vi "HEWH Staged Proportioning Valve Opening.vi"(8 "Error In":errorcluster, 10 "Elapsed Time (sec) in":dbl, 11 "Core HEWH Data Station A":T1 {"Test Patten Setup"."PRAT/RLT Sequence"."Time" format="%<%H:%M:%S>t"; "Test Patten Setup"."Total Gallons Schedule" format="%.2f"}) -> (0 "Error Out":errorcluster, 3 "Prop Valve Setting":dbl)   [LabVIEW 2016]
uses:
  Type Definitions/HEWH Output Information.ctl
  Type Definitions/HEWH Draw Pattern Setup.ctl
  Type Definitions/PRAT Test.ctl
  Utility/Save File/File Setup (Public)/Type Definition/Save File HEWH Heating Control Mode.ctl
  Draw Water Specific/Type Definitions/Terminate Draw Conditions.ctl
  Type Definitions/HEWH Start Conditions.ctl
  Draw Water Specific/Type Definitions/Check Special Condtions.ctl
  Draw Water Specific/Type Definitions/HEWH Special Condition Check.ctl
  Type Definitions/HEWH Draw Flag ENUM.ctl
  Type Definitions/HEWH Specific DAQ.ctl
  Type Definitions/HEWH Power Data.ctl
  Type Definitions/HEWH Power Elements.ctl
  Utility/Type Definitions/UTILITY Power Analyzer.ctl
  Type Definitions/HEWH Calc and Calibration.ctl
  Utility/Save File/File Setup (Public)/Type Definition/Save File DOE LabView Program.ctl
  Custom Instrument Control/MW100/Type Definitions/Station ID Selector.ctl
  Utility/Save File/File Setup.lvlib
panel:
  # "Draw Pattern Setup (24 Hour)"
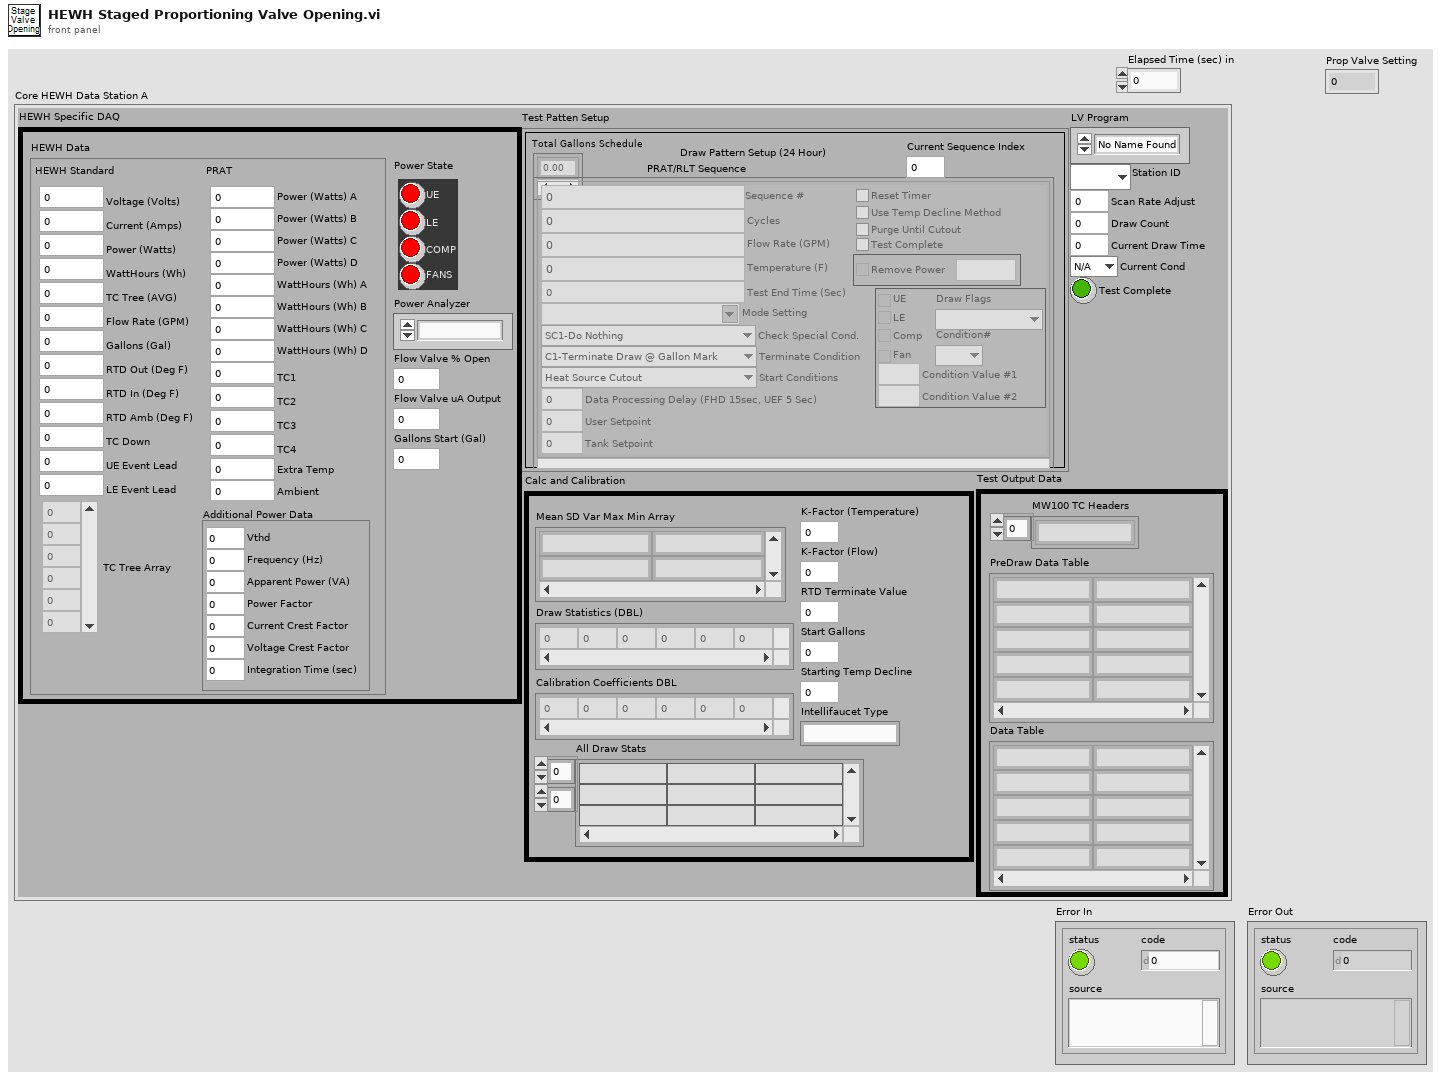
[diagram p1: front panel]
types:
  T1 = typedef "HEWH Output Information.ctl" = cluster{"Scan Rate Adjust":dbl, "Draw Count":i32, "Test Patten Setup":T2, "HEWH Specific DAQ":T10, "Test Output Data":cluster{"PreDraw Data Table":string[][], "Data Table":string[][], "MW100 TC Headers":string[]}, "Calc and Calibration":T14, "Current Draw Time":dbl, "LV Program":T15, "Station ID":T16, "Current Cond":T8, "Test Complete":bool}
  T2 = typedef "HEWH Draw Pattern Setup.ctl" = cluster{"Total Gallons Schedule":dbl[], "PRAT/RLT Sequence":T3[], "Current Sequence Index":i32}
  T3 = typedef "PRAT Test.ctl" = cluster{"Sequence #":dbl, "Cycles":i32, "Mode Setting":T4, "Flow Rate (GPM)":dbl, "Temperature (F)":dbl, "Reset Timer":bool, "Use Temp Decline Method":bool, "Terminate Condition":T5, "Condition Value #1":dbl, "UE":bool, "LE":bool, "Comp":bool, "Fan":bool, "Test End Time (Sec)":dbl, "Purge Until Cutout":bool, "Start Conditions":T6, "Condition Value #2":dbl, "Remove Power":bool, "Time":dbl, "Check Special Cond.":T7, "Condition#":T8, "Draw Flags":T9, "Data Processing Delay (FHD 15sec, UEF 5 Sec)":dbl, "Test Complete":bool, "User Setpoint":dbl, "Tank Setpoint":dbl}
  T4 = typedef "File Setup.lvlib/Save File HEWH Heating Control Mode.ctl" = string
  T5 = typedef "Terminate Draw Conditions.ctl" = enum16{"C1-Terminate Draw @ Gallon Mark", "C2-Special Last Draw (HU Test)", "C3-RTD Out <=", "C4-Mean Tank Temp <=", "C5-Decrease RTD Out (Deg F)", "C6-Time (Seconds)", "C7-Until Any Heat Source", "C8-Specific Heat Source", "C9-Do Nothing"}
  T6 = typedef "HEWH Start Conditions.ctl" = enum16{"Heat Source Cutout", "At Time (Seconds)", "Every X (Seconds)", "T2 >= X° Below Setpoint", "Seconds From Complete", "Wait for LE & Comp Cutout", "Wait for Comp Cutout", "Wait for LE Cutout", "Wait for UE Cutout"}
  T7 = typedef "Check Special Condtions.ctl" = enum16{"SC1-Do Nothing", "SC2-Check Heat Source (On-C2/Off-C1)", "SC3-Check Skip Condition", "SC4-Check Heat Source ON/Fail"}
  T8 = typedef "HEWH Special Condition Check.ctl" = enum16{"N/A", "C1", "C2", "Reset/Fail", "Skip Draw Sequence"}
  T9 = typedef "HEWH Draw Flag ENUM.ctl" = enum16{"N/A", "None(0)", "Sml(1)", "Med(2)", "SmlMed(3)", "Lrg(4)", "SmlLrg(5)", "MedLrg(6)", "SmlMedLrg(7)"}
  T10 = typedef "HEWH Specific DAQ.ctl" = cluster{"HEWH Data":T11, "Flow Valve % Open":dbl, "Power State":T12, "Power Analyzer":T13, "Flow Valve uA Output":i32, "Gallons Start (Gal)":dbl}
  T11 = typedef "HEWH Power Data.ctl" = cluster{"HEWH Standard":cluster{"Voltage (Volts)":dbl, "Current (Amps)":dbl, "Power (Watts)":dbl, "WattHours (Wh)":dbl, "TC Tree (AVG)":dbl, "Flow Rate (GPM)":dbl, "Gallons (Gal)":dbl, "RTD Out (Deg F)":dbl, "RTD In (Deg F)":dbl, "RTD Amb (Deg F)":dbl, "TC Down":dbl, "UE Event Lead":i32, "LE Event Lead":i32, "TC Tree Array":dbl[]}, "PRAT":cluster{"Power (Watts) A":dbl, "Power (Watts) B":dbl, "Power (Watts) C":dbl, "Power (Watts) D":dbl, "TC1":dbl, "TC2":dbl, "TC3":dbl, "TC4":dbl, "WattHours (Wh) A":dbl, "WattHours (Wh) B":dbl, "WattHours (Wh) C":dbl, "WattHours (Wh) D":dbl, "Ambient":dbl, "Extra Temp":dbl}, "Additional Power Data":cluster{"Vthd":dbl, "Frequency (Hz)":dbl, "Apparent Power (VA)":dbl, "Power Factor":dbl, "Current Crest Factor":dbl, "Voltage Crest Factor":dbl, "Integration Time (sec)":dbl}}
  T12 = typedef "HEWH Power Elements.ctl" = cluster{"UE":bool, "LE":bool, "COMP":bool, "FANS":bool}
  T13 = typedef "UTILITY Power Analyzer.ctl" = enum16{"", "APLUS", "WT210", "WT500", "WT300", "OSI", "Debug", "WT230", "WT300_1", "WT300_2"}
  T14 = typedef "HEWH Calc and Calibration.ctl" = cluster{"Mean SD Var Max Min Array":string[][], "Draw Statistics (DBL)":dbl[][], "Calibration Coefficients DBL":dbl[][], "Start Gallons":dbl, "Starting Temp Decline":dbl, "K-Factor (Temperature)":dbl, "All Draw Stats":string[][], "RTD Terminate Value":dbl, "K-Factor (Flow)":dbl, "Intellifaucet Type":string}
  T15 = typedef "File Setup.lvlib/Save File DOE LabView Program.ctl" = enum16{"No Name Found", "DOE Stand", "Dishwasher Kitchen", "Portable Stand", "HEWH", "Dryer", "Dryer WILT", "HCC", "PRAT", "HEWH RLT", "Refrigeration"}
  T16 = typedef "Station ID Selector.ctl" = enum16{"", "A", "B", "C", "D", "Global"}
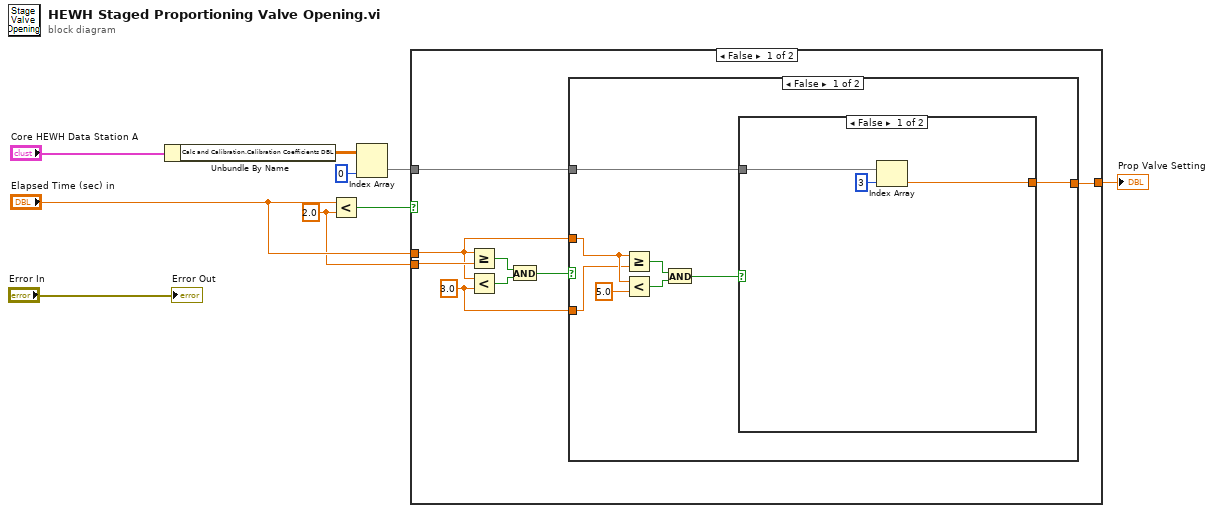
[diagram p0: block diagram]
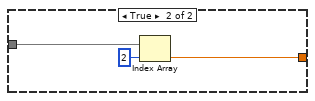
[diagram p2: hidden frame]
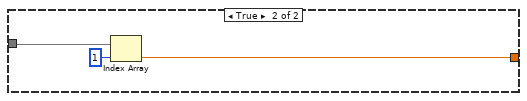
[diagram p3: hidden frame]
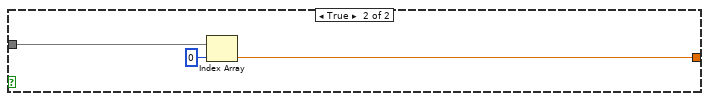
[diagram p4: hidden frame]
diagram:
  w5 = 2.0 ("y")
  n1 = Unbundle By Name("Core HEWH Data Station A") -> ("Calc and Calibration.Calibration Coefficients DBL"=w4:dbl[][])
  n2 = Less?(x="Elapsed Time (sec) in", y=w5) -> (x < y?=w7:bool)
  n3 = Index Array(array=w4, index (col)=0 ("disabled index (col)")) -> (element=w2:dbl[])  [unwired: 1 in]
  n4 = case shown="False" w7 {
    tunnel: "Elapsed Time (sec) in" -> [w11 _]
    tunnel: w5 -> [w14 _]
    tunnel: w2 -> [w13 w37]
    tunnel: [w12 w35] -> w1
    frame False {
      w10 = 3.0 ("y")
      n5 = Greater Or Equal?(x=w11, y=w14) -> (x >= y?=w17:bool)
      n6 = Less?(x=w11, y=w10) -> (x < y?=w16:bool)
      n7 = And(x=w17, y=w16) -> (x .and. y?=w15:bool)
      n8 = case shown="False" w15 {
        tunnel: w13 -> [w19 w33]
        tunnel: [w18 w32] -> w12
        tunnel: w11 -> [w22 _]
        tunnel: w10 -> [w21 _]
        frame False {
          n9 = Greater Or Equal?(x=w22, y=w21) -> (x >= y?=w23:bool)
          n10 = Less?(x=w22, y=5.0) -> (x < y?=w24:bool)
          n11 = And(x=w23, y=w24) -> (x .and. y?=w20:bool)
          n12 = case shown="False" w20 {
            tunnel: w19 -> [w27 w30]
            tunnel: [w26 w29] -> w18
            frame False {
              n13 = Index Array(array=w27, index=3) -> (element=w26:dbl)
            }
            frame True {
              n14 = Index Array(array=w30, index=2) -> (element=w29:dbl)
            }
          }
        }
        frame True {
          n15 = Index Array(array=w33, index=1) -> (element=w32:dbl)
        }
      }
    }
    frame True {
      n16 = Index Array(array=w37, index=0) -> (element=w35:dbl)
    }
  }
  "Prop Valve Setting" <- w1
  "Error Out" <- "Error In"
